vi "Configure SMU Current Slew Rate.vi"(7 "Enable Current Slew Rate Override (False)":bool, 8 "error in (no error)":errorcluster {"code" format="%.0x"}, 9 "Current Slew Rate (9.9E+37 A/s)":dbl=9.9e+37 format="%^.3e", 10 "Channel Name (1)":string="1", 11 "VISA resource name":refnum<visa-resource-name>) -> (0 "error out":errorcluster {"code" format="%.0x"}, 3 "VISA resource name out":refnum<visa-resource-name>)   [LabVIEW 2016, in "Agilent N6700 Series.lvlib"]
doc: "Sets the current slew rate.\n\n<b>Note:</b>\nThis VI only applies to model N678xA SMU and N679xA."
uses:
  <instrlib>/Agilent N6700 Series/Agilent N6700 Series.lvlib
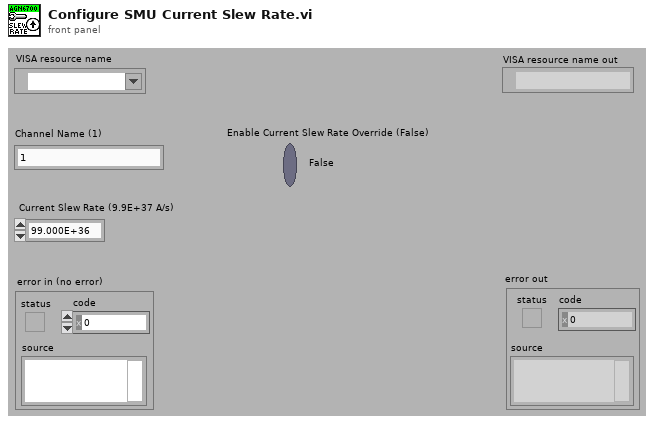
[diagram p1: front panel]
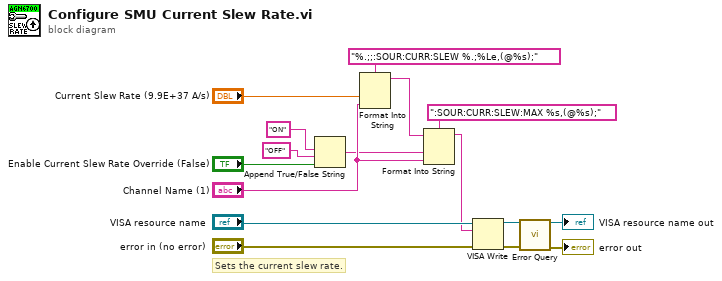
[diagram p0: block diagram]
diagram:
  # "Sets the current slew rate."
  n1 = Append True/False String(1:"Enable Current Slew Rate Override (False)", 2:"OFF", 3:"ON") -> (0:w3:string)  [unwired: 1 in]
  n2 = Format Into String(format string="%.;;:SOUR:CURR:SLEW %.;%Le,(@%s);", "Current Slew Rate (9.9E+37 A/s)", "Channel Name (1)") -> (resulting string=w6:string)  [unwired: 2 in, 1 out]
  n3 = Format Into String(format string=":SOUR:CURR:SLEW:MAX %s,(@%s);", initial string=w6, w3, "Channel Name (1)") -> (resulting string=w9:string)  [unwired: 1 in, 1 out]
  n4 = VISA Write(VISA resource name="VISA resource name", write buffer=w9, error in (no error)="error in (no error)") -> (VISA resource name out=w12:refnum<visa-resource-name>, error out=w11:errorcluster)  [unwired: 1 out]
  n5 = call <instrlib>:"Error Query.vi"("VISA resource name"=w12, "error in (no error)"=w11) -> ("VISA resource name out"=→"VISA resource name out":refnum<visa-resource-name>, "error out"=→"error out":errorcluster)  [unwired: 10 in, 2 out]
